vi "LEP_RV_BuildSpec_CompileOptionsDlg.vi"(8 "error in (no error)":errorcluster, 10 "page sync rendezvous":T2, 11 "Close Event":refnum<user-event>) -> ()   [LabVIEW 2011]
doc: "Specifies advanced code generation options."
uses:
  resource/dialog/PreferencesDialog/optionsFrame_EventData1.ctl
  resource/dialog/PreferencesDialog/optionsFrame_PageInitData.ctl
  <vilib>/Platform/EmbProject/Plugins/utilities/LEP_Utilities_GetSetProjectData_Variant.vi
panel:
  in  "Use MicroLib":bool
  in  "Optimize heap size":bool
  out "Build settings conflicts":i32(listbox)=1
  in  "Enable cross-module optimization":bool
  in  "Include paths":path[](array[path])
  in  "Optimize for time":bool
  in  "Optimization":u16(ring)=2 items=["Level 0 (-O0)", "Level 1 (-O1)", "Level 2 (-O2)", "Level 3 (-O3)"]
  in  "Mode":u16(ring)=1 items=["ARM-Mode", "Thumb-Mode"]
  in  "Extra linker flags":string
  in  "Extra compiler flags":string
  in  "Preprocessor symbols (define)":string
  in  "Page VI Init Data":T1
  in  "error msg format string":string="There was a problem applying the options from the %s category. The error message is \"%s.\""
  # "Build options"
  # "Advanced Code Generation Options"
  # "Debug options"
  # "Memory options"
  # "Run-time options"
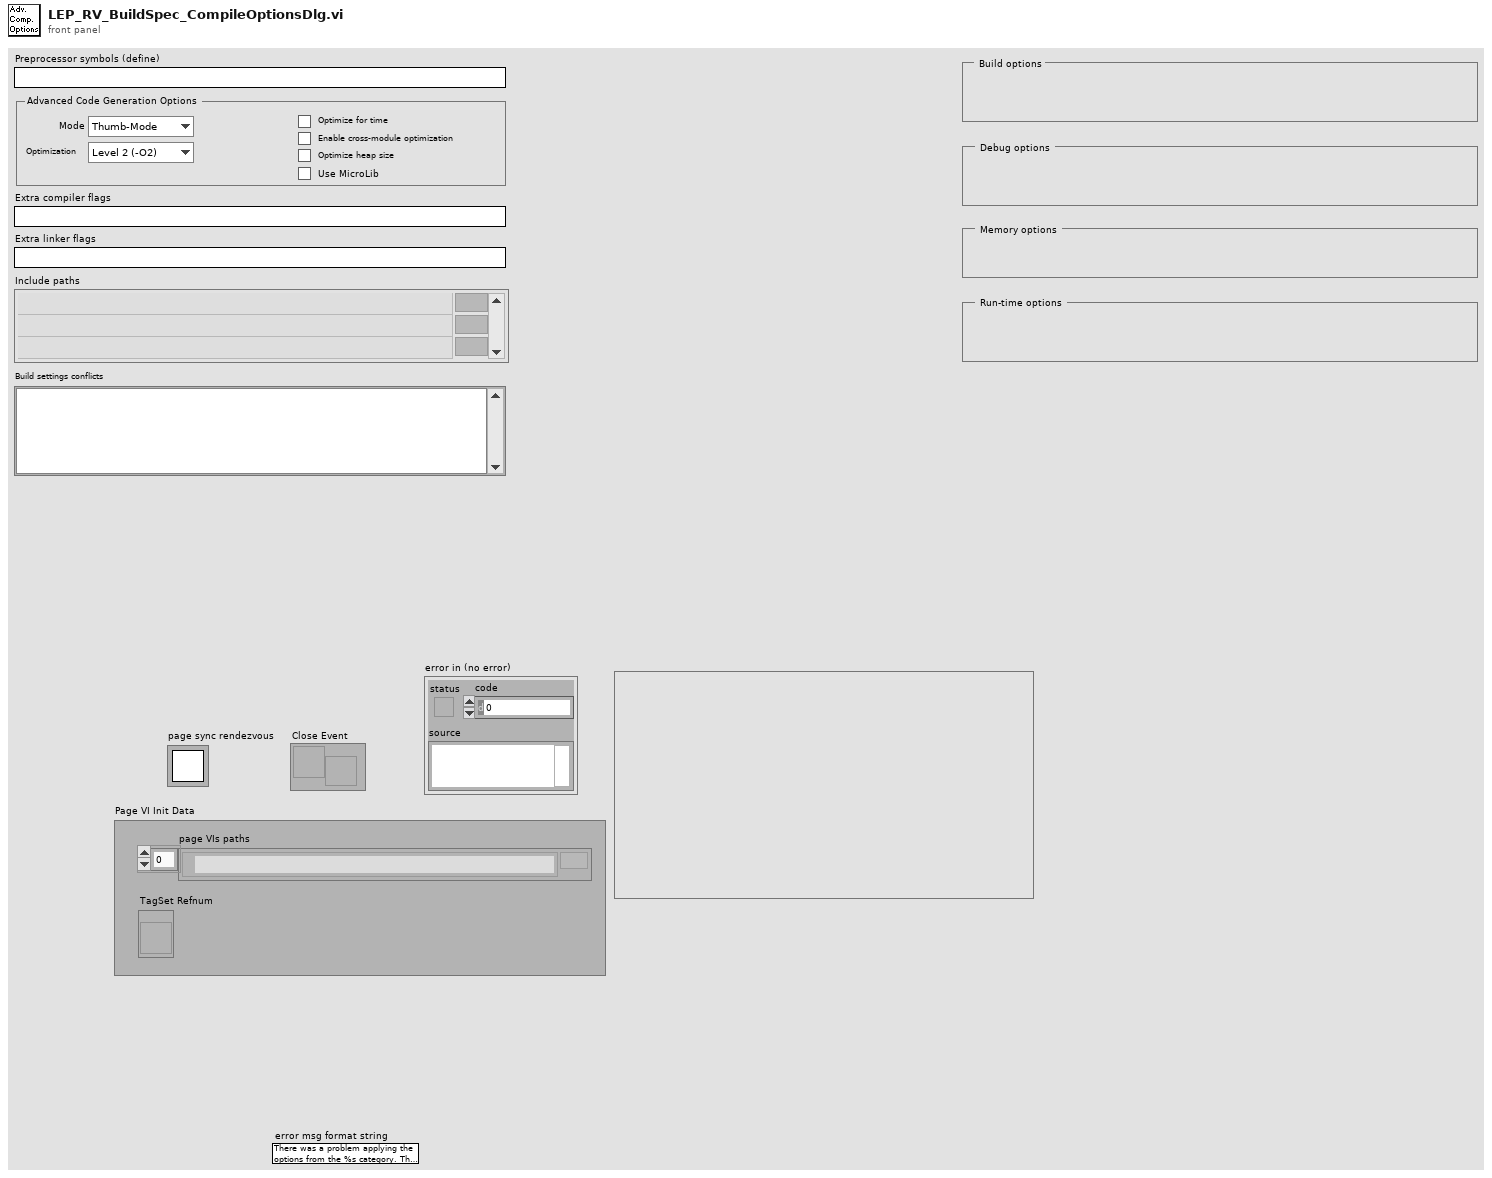
[diagram p1: front panel]
types:
  T1 = typedef "optionsFrame_PageInitData.ctl" = cluster{"page VIs paths":path[], "TagSet Refnum":refnum<vi>}
  T2 = typedef "Rendezvous RefNum" = refnum<k1>
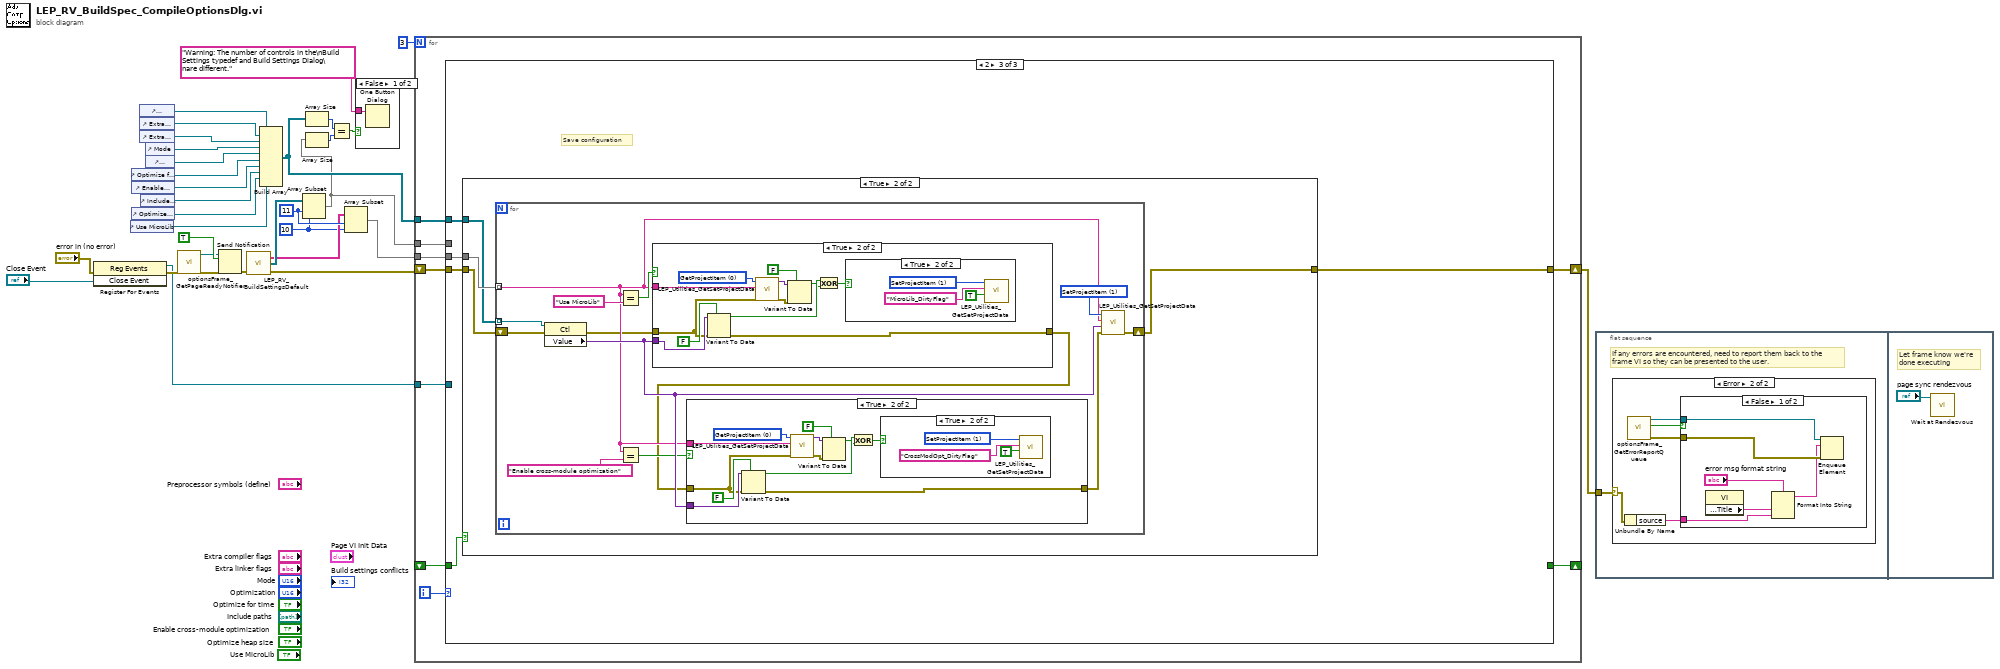
[diagram p0: block diagram]
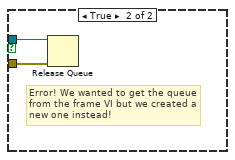
[diagram p3: hidden frame]
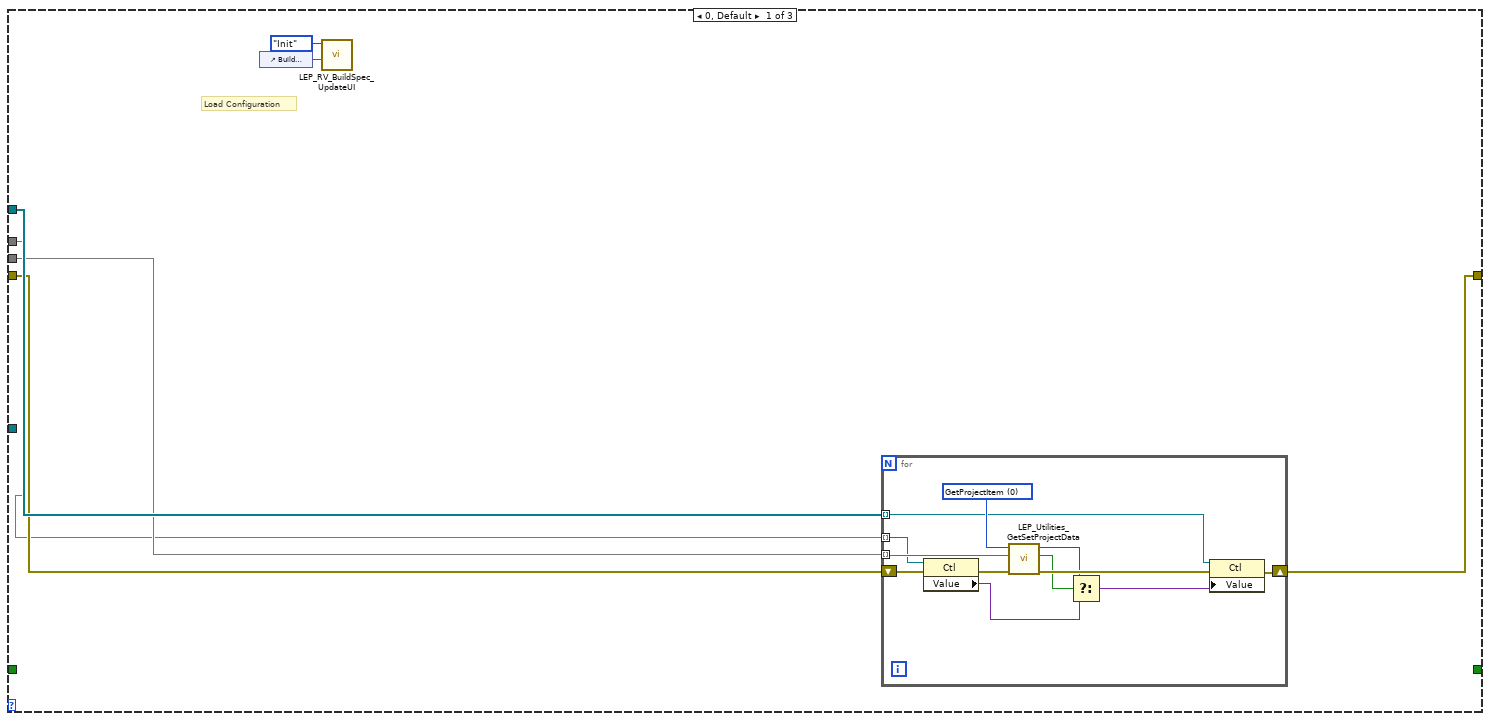
[diagram p5: hidden frame]
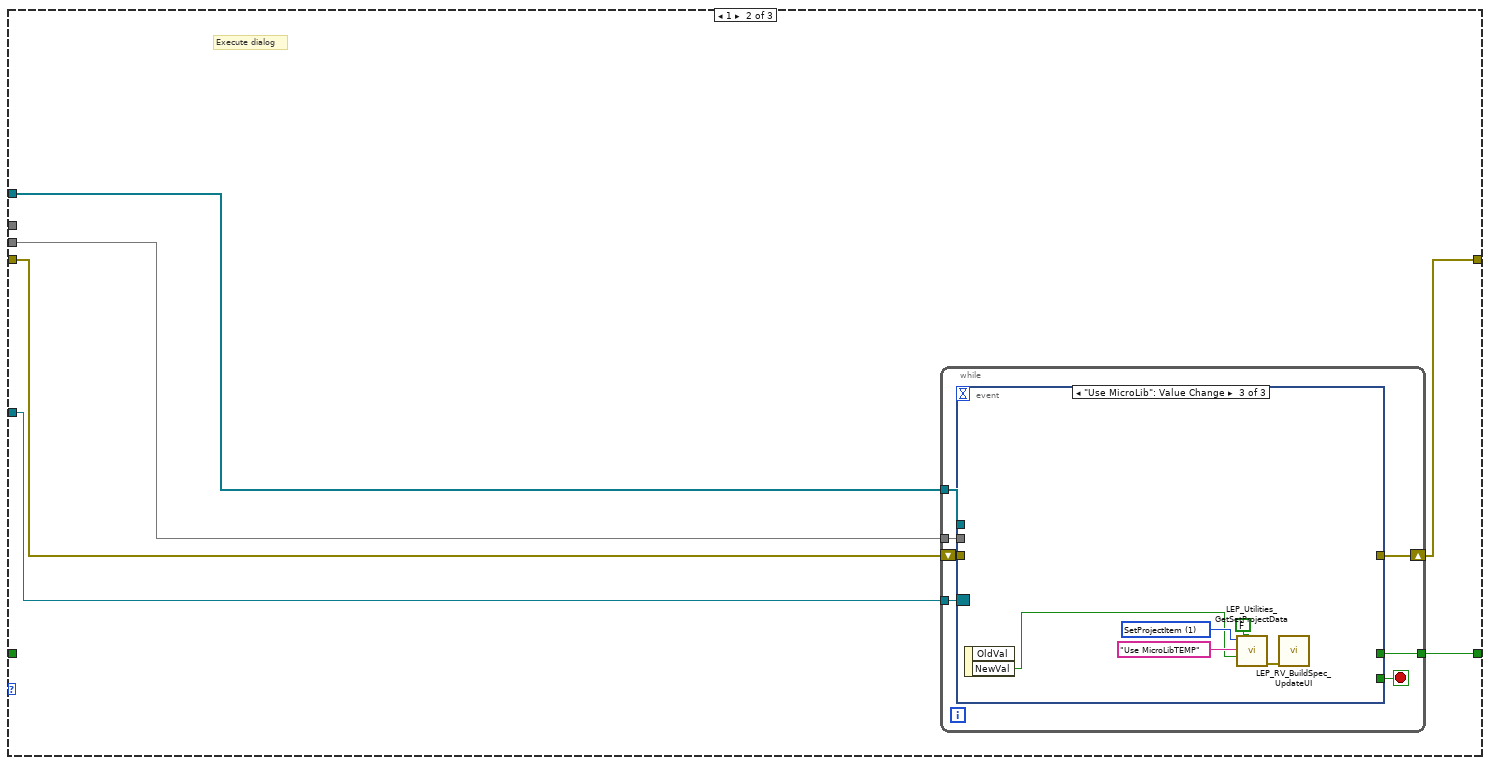
[diagram p6: hidden frame]
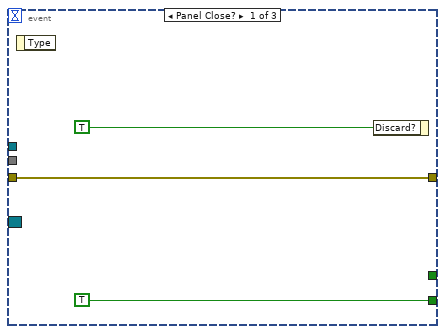
[diagram p7: hidden frame]
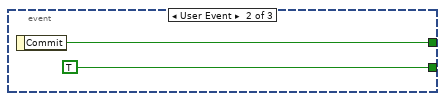
[diagram p8: hidden frame]
diagram:
  w6 = 10 ("length")
  w12 = 11 ("index")
  n1 = register-events(error in="error in (no error)", "Close Event") -> (reference out=w18:refnum<event-registration>, error out=w21:errorcluster)  [unwired: 1 in]
  n2 = control-ref of="Use MicroLib"() -> (w1:refnum<vi>)
  n3 = control-ref of="Optimize for time"() -> (w14:refnum<vi>)
  n4 = control-ref of="Enable cross-module optimization"() -> (w3:refnum<vi>)
  n5 = control-ref of="Optimize heap size"() -> (w2:refnum<vi>)
  n6 = control-ref of="Preprocessor symbols (define)"() -> (w7:refnum<vi>)
  n7 = control-ref of="Extra compiler flags"() -> (w9:refnum<vi>)
  n8 = control-ref of="Extra linker flags"() -> (w8:refnum<vi>)
  n9 = control-ref of="Include paths"() -> (w4:refnum<vi>)
  n10 = control-ref of="Mode"() -> (w16:refnum<vi>)
  n11 = control-ref of="Optimization"() -> (w15:refnum<vi>)
  n12 = call "optionsFrame_GetPageReadyNotifier.vi"("error in (no error)"=w21) -> ("error out"=w20:errorcluster, "notifier out"=w22:refnum<notifier>)  [unwired: 9 out]
  n13 = Send Notification(notification=TRUE, notifier=w22, error in (no error)=w20) -> (error out=w19:errorcluster)  [unwired: 1 out]
  n14 = call "LEP_RV_BuildSettingsDefault.vi"("error in (no error)"=w19) -> ("error out"=w31:errorcluster, "Default Values"=w13:refnum<vi>[], "Attribute Name"=w11:string[])  [unwired: 2 out]
  n15 = Build Array(w7, w9, w8, w16, w15, w14, w3, w4, w2, w1) -> (w27:refnum<vi>[])
  n16 = Array Subset(array=w13, index=w12, length=w6) -> (w5:refnum<vi>[])
  n17 = Array Size(array=w27) -> (size(s)=w29:i32)
  n18 = Array Size(array=w5) -> (size(s)=w30:i32)
  n19 = Equal?(x=w29, y=w30) -> (x = y?=w28:bool)
  n20 = Array Subset(array=w11, index=w12, length=w6) -> (w10:string[])
  n21 = case shown="False" w28 {
    tunnel: "Warning: The number of controls in the\nBuild Settings typedef and Build Settings Dialog\nare different." -> [w33 _]
    frame False {
      n22 = One Button Dialog(message=w33) -> ()  [unwired: 2 out]
    }
    frame True {
    }
  }
  n23 = for {
    N: 3 -> [_]
    shift-right: [w40] -> w17
    shift-left: w31 -> [w41]
    shift-right: [w39] -> _
    shift-left: _ -> [w38]
    tunnel: w27 -> [w37]
    tunnel: w10 -> [w36]
    tunnel: w5 -> [w35]
    tunnel: w18 -> [w34]
    i -> [w42]
    n24 = case shown="2" w42 {
      tunnel: w41 -> [w48 w67 w88]
      tunnel: [w47 w66 w87] -> w40
      tunnel: [_ w65 _] -> w39
      tunnel: w38 -> [_ _ w89]
      tunnel: w37 -> [w49 w63 w85]
      tunnel: w36 -> [w46 w64 w86]
      tunnel: w35 -> [w45 _ _]
      tunnel: w34 -> [_ w62 _]
      frame 0, Default {
        # "Load Configuration"
        n25 = control-ref of="Build settings conflicts"() -> (w43:refnum<vi>)
        n26 = call "LEP_RV_BuildSpec_UpdateUI.vi"("Build conflicts ref"=w43, "Action"=enum16{"Init", "UpdateUI"}."Init") -> ()  [unwired: 2 in, 8 out]
        n27 = for {
          tunnel: w49 -> [w50] mode=indexing
          shift-right: [w59] -> w47
          shift-left: w48 -> [w57]
          tunnel: w46 -> [w58] mode=indexing
          tunnel: w45 -> [w55] mode=indexing
          w61 = u16 0 items=["GetProjectItem", "SetProjectItem"] ("Command")
          n28 = property class="Ctl"(reference=w55, error in=w57) -> (error out=w56:errorcluster, "Value"=w51:variant)  [unwired: 1 out]
          n29 = call-poly <vilib>:"LEP_Utilities_GetSetProjectData.vi"("error in"=w56, "ItemName"=w58, "Command"=w61) -> ("error out"=w60:errorcluster, "Found/Replaced?"=w52:bool, "Variant Out"=w53:variant)  [unwired: 2 in, 4 out]
          n30 = Select(t=w53, s=w52, f=w51) -> (s? t:f=w54:variant)
          n31 = property class="Ctl"(reference=w50, error in=w60, "Value"=w54) -> (error out=w59:errorcluster)  [unwired: 1 out]
        }
      }
      frame 1 {
        # "Execute dialog"
        n32 = while {
          shift-right: [w73] -> w66
          shift-left: w67 -> [w74]
          tunnel: [w72] -> w65
          tunnel: w64 -> [w70]
          tunnel: w63 -> [w69]
          tunnel: w62 -> [w68]
          stop <- w71 stop-if-true
          n33 = event shown="[2] \"Use MicroLib\": Value Change" {
            selector: w68 -> [_ _ _]
            dyn-events: _ -> [_ _ _]
            timeout: _ -> [_ _ _]
            tunnel: w74 -> [w76 _ _]
            tunnel: [w76 _ _] -> w73
            tunnel: [_ w78 _] -> w72
            tunnel: [TRUE TRUE ("Cancel") _] -> w71
            tunnel: w70 -> [_ _ _]
            tunnel: w69 -> [_ _ _]
            event Panel Close? {
              n34 = event-data() -> ()  [unwired: 2 out]
              n35 = event-data("Discard?"=TRUE) -> ()  [unwired: 1 in, 1 out]
            }
            event User Event {
              n36 = event-data() -> ("Commit"=w78:bool)  [unwired: 1 out]
            }
            event "Use MicroLib": Value Change {
              w84 = u16 1 items=["GetProjectItem", "SetProjectItem"] ("Command")
              n37 = event-data() -> ("NewVal"=w81:bool)  [unwired: 2 out]
              n38 = call-poly <vilib>:"LEP_Utilities_GetSetProjectData.vi"("Is Persistent"=FALSE, "Variant In"=w81, "ItemName"="Use MicroLibTEMP", "Command"=w84) -> ("error out"=w80:errorcluster)  [unwired: 2 in, 5 out]
              n39 = call "LEP_RV_BuildSpec_UpdateUI.vi"("error in (no error)"=w80) -> ()  [unwired: 3 in, 8 out]
            }
          }
        }
      }
      frame 2 {
        # "Save configuration"
        n40 = case shown="True" w89 {
          tunnel: w88 -> [w90 w94]
          tunnel: [w90 w91] -> w87
          tunnel: w86 -> [_ w93]
          tunnel: w85 -> [_ w92]
          frame False {
          }
          frame True {
            n41 = for {
              shift-right: [w105] -> w91
              shift-left: w94 -> [w106]
              tunnel: w93 -> [w99] mode=indexing
              tunnel: w92 -> [w103] mode=indexing
              w107 = u16 1 items=["GetProjectItem", "SetProjectItem"] ("Command")
              n42 = property class="Ctl"(reference=w103, error in=w106) -> (error out=w97:errorcluster, "Value"=w100:variant)  [unwired: 1 out]
              n43 = Equal?(x=w99, y="Enable cross-module optimization" ("x")) -> (x = y?=w98:bool)
              n44 = Equal?(x=w99, y="Use MicroLib" ("x")) -> (x = y?=w104:bool)
              n45 = case shown="True" w104 {
                tunnel: w99 -> [_ w136]
                tunnel: w100 -> [_ w132]
                tunnel: w97 -> [w124 w126]
                tunnel: [w124 w127] -> w96
                frame False {
                }
                frame True {
                  w135 = u16 0 items=["GetProjectItem", "SetProjectItem"] ("Command")
                  n46 = Variant To Data(error in=w126, type=FALSE, Variant=w132) -> (data=w130:bool, error out=w127:errorcluster)
                  n47 = call-poly <vilib>:"LEP_Utilities_GetSetProjectData.vi"("error in"=w126, "ItemName"=w136, "Command"=w135) -> ("error out"=w134:errorcluster, "Variant Out"=w133:variant)  [unwired: 2 in, 5 out]
                  n48 = Variant To Data(error in=w134, type=FALSE, Variant=w133) -> (data=w128:bool)  [unwired: 1 out]
                  n49 = Exclusive Or(1:w128, 2:w130) -> (0:w125:bool)
                  n50 = case shown="True" w125 {
                    frame False {
                    }
                    frame True {
                      w139 = u16 1 items=["GetProjectItem", "SetProjectItem"] ("Command")
                      n51 = call-poly <vilib>:"LEP_Utilities_GetSetProjectData.vi"("Variant In"=TRUE, "ItemName"="MicroLib_DirtyFlag", "Command"=w139) -> ()  [unwired: 2 in, 7 out]
                    }
                  }
                }
              }
              n52 = case shown="True" w98 {
                tunnel: w99 -> [_ w120]
                tunnel: w100 -> [_ w116]
                tunnel: w96 -> [w108 w110]
                tunnel: [w108 w111] -> w95
                frame False {
                }
                frame True {
                  w119 = u16 0 items=["GetProjectItem", "SetProjectItem"] ("Command")
                  n53 = Variant To Data(error in=w110, type=FALSE, Variant=w116) -> (data=w114:bool, error out=w111:errorcluster)
                  n54 = call-poly <vilib>:"LEP_Utilities_GetSetProjectData.vi"("error in"=w110, "ItemName"=w120, "Command"=w119) -> ("error out"=w118:errorcluster, "Variant Out"=w117:variant)  [unwired: 2 in, 5 out]
                  n55 = Variant To Data(error in=w118, type=FALSE, Variant=w117) -> (data=w112:bool)  [unwired: 1 out]
                  n56 = Exclusive Or(1:w112, 2:w114) -> (0:w109:bool)
                  n57 = case shown="True" w109 {
                    frame False {
                    }
                    frame True {
                      w123 = u16 1 items=["GetProjectItem", "SetProjectItem"] ("Command")
                      n58 = call-poly <vilib>:"LEP_Utilities_GetSetProjectData.vi"("Variant In"=TRUE, "ItemName"="CrossModOpt_DirtyFlag", "Command"=w123) -> ()  [unwired: 2 in, 7 out]
                    }
                  }
                }
              }
              n59 = call-poly <vilib>:"LEP_Utilities_GetSetProjectData.vi"("error in"=w95, "Variant In"=w100, "ItemName"=w99, "Command"=w107) -> ("error out"=w105:errorcluster)  [unwired: 1 in, 6 out]
            }
          }
        }
      }
    }
  }
  n60 = flat-sequence {
    tunnel: w17 -> [w140]
    frame #0 {
      # "If any errors are encountered, need to report them back to the \nframe VI so they can be presented to the user."
      n61 = case shown="Error" w140 {
        selector: w140 -> [_ w142]
        frame No Error {
        }
        frame Error {
          n62 = Unbundle By Name(w142) -> ("source"=w141:string)
          n63 = call "optionsFrame_GetErrorReportQueue.vi"() -> ("error out"=w143:errorcluster, "created new?"=w145:bool, "queue out"=w144:refnum<queue>)  [unwired: 9 out]
          n64 = case shown="False" w145 {
            tunnel: w144 -> [w151 w153]
            tunnel: w143 -> [w150 w152]
            tunnel: w141 -> [w147 _]
            frame False {
              n65 = property class="VI"() -> ("Front Panel.Title"=w148:string)  [unwired: 2 in, 2 out]
              n66 = Format Into String(format string="error msg format string", w148, w147) -> (resulting string=w146:string)  [unwired: 2 in, 1 out]
              n67 = Enqueue Element(queue=w151, element=w146, error in (no error)=w150) -> ()  [unwired: 4 out]
            }
            frame True {
              # "Error! We wanted to get the queue\nfrom the frame VI but we created a\nnew one instead!"
              n68 = Release Queue(queue=w153, error in (no error)=w152) -> ()  [unwired: 4 out]
            }
          }
        }
      }
    }
    frame #1 {
      # "Let frame know we're \ndone executing"
      n69 = call <vilib>:"Wait at Rendezvous.vi"("rendezvous"="page sync rendezvous") -> ()  [unwired: 2 in, 5 out]
    }
  }
